vi "test - filename pure English.vi"(8 "error in (no error)":errorcluster, 11 "TestCase in":refnum<class "testcase-documentation.lvclass">) -> (0 "error out":errorcluster, 3 "TestCase out":refnum<class "testcase-documentation.lvclass">)   [LabVIEW 2017, in "testcase-documentation.lvclass"]
uses:
  testcase-documentation.lvclass
  <vilib>/addons/_JKI Toolkits/VI Tester/TestCase.llb/TestCase.lvclass
  src/user.lib/_NEVSTOP/Communicable State Machine(CSM)/_Shared/CSM Shared.lvlib
  src/user.lib/_NEVSTOP/Communicable State Machine(CSM)/Communicable State Machine.lvlib
  C:/Program Files (x86)/National Instruments/LabVIEW 2017/vi.lib/addons/_JKI Toolkits/VI Tester/TestCase.llb/TestCase.lvclass
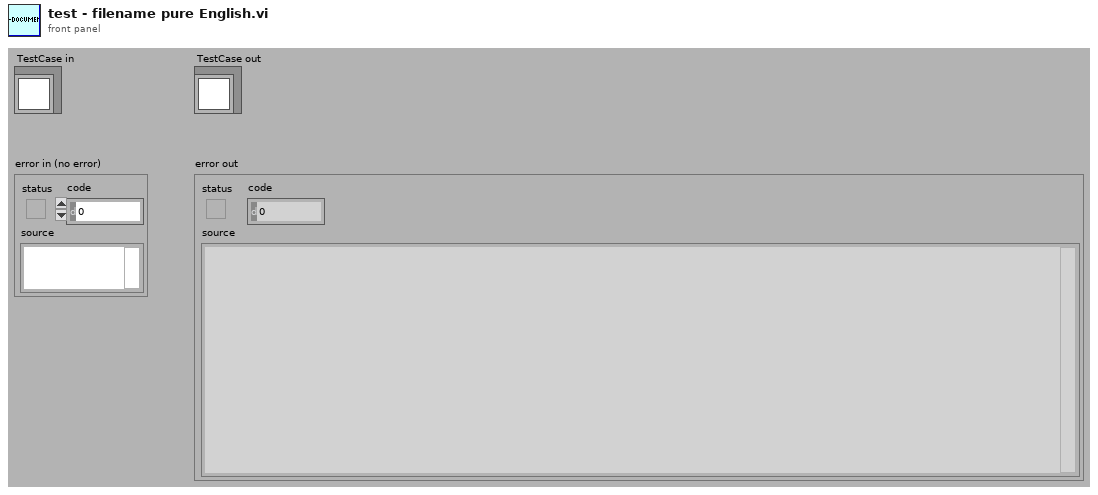
[diagram p1: front panel]
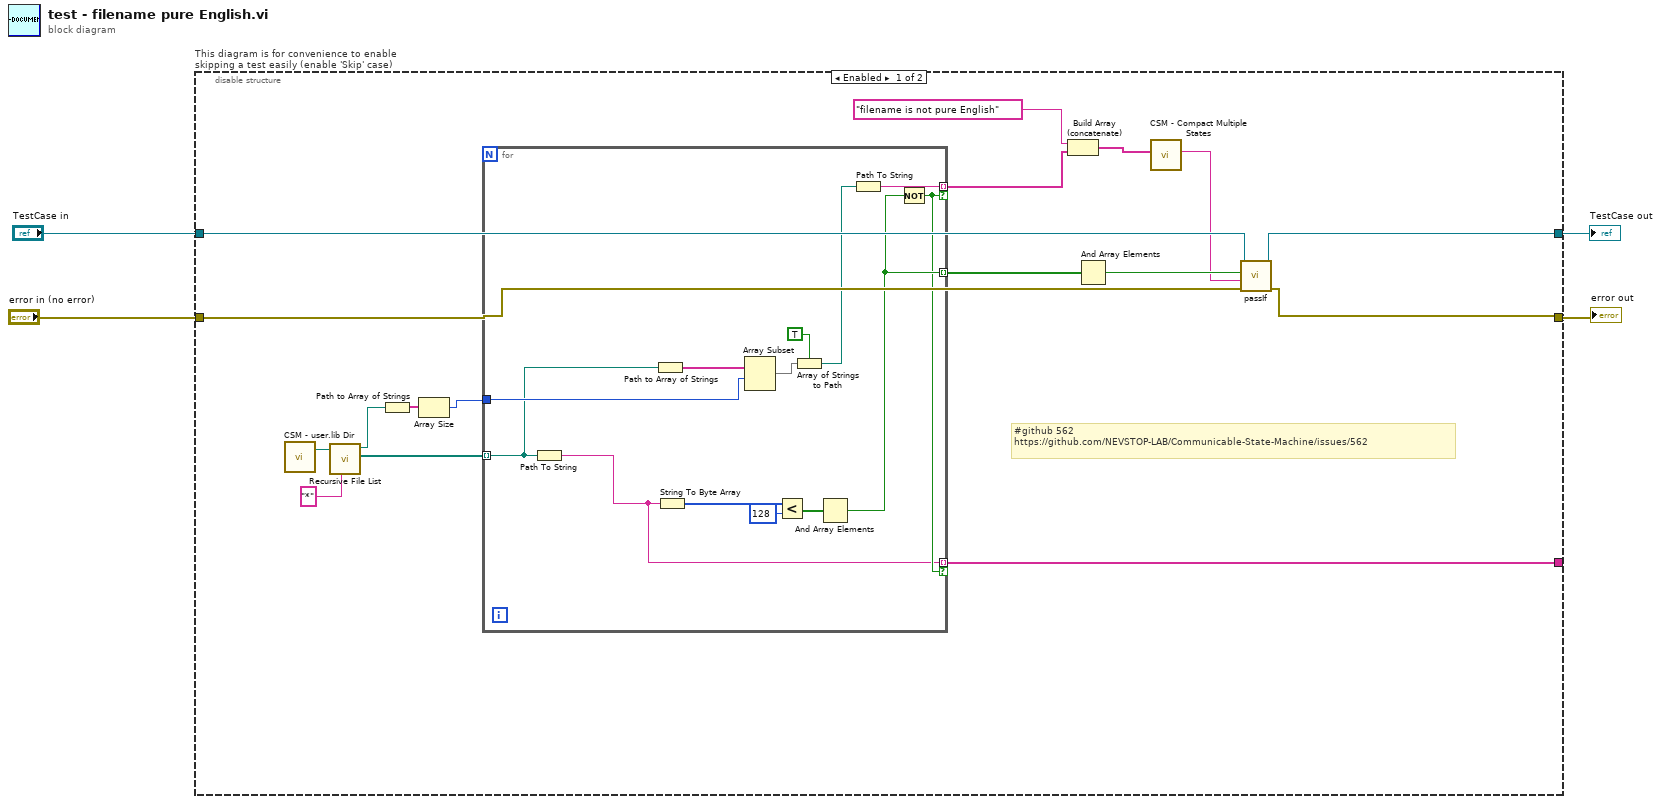
[diagram p0: block diagram]
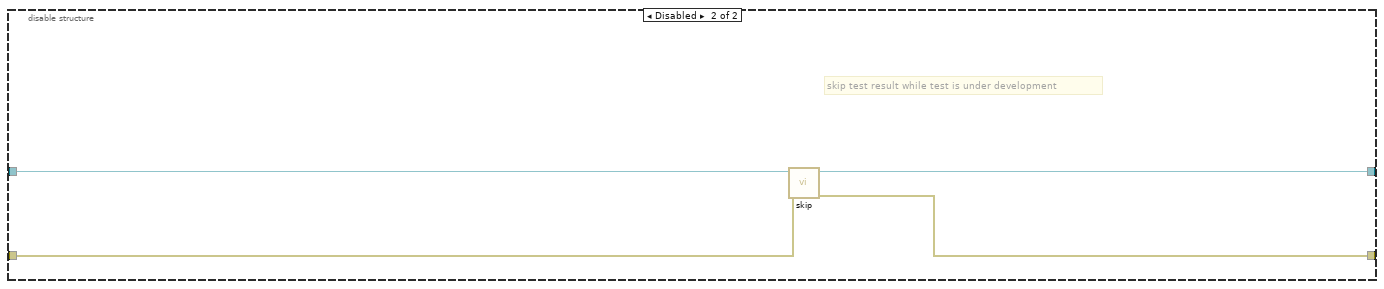
[diagram p2: hidden frame]
diagram:
  n1 = disable-structure "This diagram is for convenience to enable skipping a test easily (enable 'Skip' case)" shown="Enabled" {
    disable-tunnel: "TestCase in" -> [w21 w38]
    disable-tunnel: [w20 w36] -> w1
    disable-tunnel: [w19 w37] -> w3
    disable-tunnel: "error in (no error)" -> [w18 w35]
    disable-tunnel: [w15 _] -> _
    frame Enabled {
      # "#github 562\nhttps://github.com/NEVSTOP-LAB/Communicable-State-Machine/issues/562"
      n2 = call "CSM - user.lib Dir.vi"() -> ("csm_user.lib_dir"=w14:path)  [unwired: 2 in, 1 out]
      n3 = call <vilib>:"Recursive File List.vi"("pattern"="*", "Folder Path"=w14) -> ("All Files in Dir"=w12:path[], "dup Folder Path"=w10:path)  [unwired: 5 in, 3 out]
      n4 = Path to Array of Strings(0:w10) -> (2:w11:string[])  [unwired: 1 out]
      n5 = Array Size(array=w11) -> (size(s)=w9:i32)
      n6 = for {
        tunnel: w9 -> [w34]
        tunnel: [w25] -> w17 mode=indexing
        tunnel: [w30] -> w7 mode=indexing if=w24
        tunnel: [w23] -> w15 mode=indexing if=w24
        tunnel: w12 -> [w22] mode=indexing
        n7 = Path To String(path=w22) -> (string=w23:string)
        n8 = Path to Array of Strings(0:w22) -> (2:w27:string[])  [unwired: 1 out]
        n9 = String To Byte Array(string=w23) -> (unsigned byte array=w33:u8[])
        n10 = Array Subset(array=w27, index=w34) -> (w29:string[])  [unwired: 1 in]
        n11 = Less?(x=w33, y=u8 128) -> (x < y?=w31:bool[])
        n12 = Array of Strings to Path(0:w29, 1:TRUE ("relative")) -> (2:w26:path)
        n13 = And Array Elements(Boolean array=w31) -> (logical AND=w25:bool)
        n14 = Path To String(path=w26) -> (string=w30:string)
        n15 = Not(x=w25) -> (.not. x?=w24:bool)
      }
      n16 = Build Array (concatenate)("filename is not pure English" ("message (\"\")"), w7) -> (w8:string[])
      n17 = And Array Elements(Boolean array=w17) -> (logical AND=w16:bool)
      n18 = call "CSM - Compact Multiple States.vi"("Multiple States"=w8) -> ("States"=w5:string)  [unwired: 9 in]
      n19 = call-dynamic "passIf.vi"("error in (no error)"=w18, "message (\"\")"=w5, "pass"=w16, "TestCase in"=w21) -> ("error out"=w19:errorcluster, "TestCase out"=w20:refnum<class "testcase-documentation.lvclass">)  [unwired: 6 in]
    }
    frame Disabled {
      # "skip test result while test is under development"
      n20 = call <vilib>:"skip.vi"("error in (no error)"=w35, "TestCase in"=w38) -> ("error out"=w37:errorcluster, "TestCase out"=w36:refnum<class "testcase-documentation.lvclass">)  [unwired: 8 in]
    }
  }
  "error out" <- w3
  "TestCase out" <- w1
